vi "KepcoDCPwr Reset with Defaults.vi"(0 "VISA Session":refnum<visa-resource-name>, 5 "Model In":string, 7 "channel name (\"\")":string="\"\"", 11 "error in (no error)":errorcluster {"code" format="%.0x"}) -> (4 "VISA Session Out":refnum<visa-resource-name>, 6 "Model Out":string, 8 "channel name out (\"\")":string="\"\"" caption="channel name Out (\"\")", 15 "error out":errorcluster {"code" format="%.0x"})   [LabVIEW 2010]
doc: "This VI resets the instrument and applies initial user specified settings from the Logical Name which was used to initialize the session. If the session was created without a Logical Name, this VI is equivalent to the KepcoDCPwr Reset.vi."
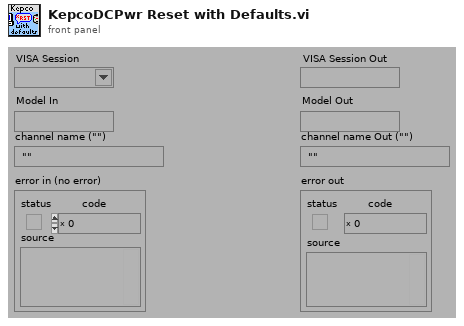
[diagram p1: front panel]
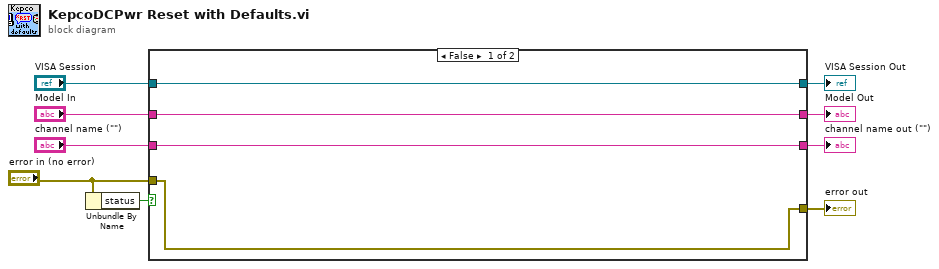
[diagram p0: block diagram]
diagram:
  n1 = Unbundle By Name("error in (no error)") -> ("status"=w8:bool)
  n2 = case shown="False" w8 {
    tunnel: [w10 w17] -> w9
    tunnel: "error in (no error)" -> [w10 w17]
    tunnel: [w13 w16] -> w3
    tunnel: "VISA Session" -> [w13 w16]
    tunnel: [w12 w15] -> w2
    tunnel: "Model In" -> [w12 w15]
    tunnel: [w11 w14] -> w1
    tunnel: "channel name (\"\")" -> [w11 w14]
    frame False {
    }
    frame True {
    }
  }
  "error out" <- w9
  "channel name out (\"\")" <- w1
  "VISA Session Out" <- w3
  "Model Out" <- w2
